vi "Helper - Overlay waypoints.vi"(11 "Refnum in":T1) -> (3 "Refnum out":T1)   [LabVIEW 2011]
uses:
  <vilib>/vision/Image Controls.llb/IMAQ Image.ctl
  2 Globals/2 Global.vi
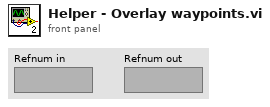
[diagram p1: front panel]
types:
  T1 = typedef "IMAQ Image.ctl" = refnum<image>
  T2 = typedef "ocuWaypoints.ctl" = cluster{"Waypoints Array":T3[], "Current Waypoint":dbl}
  T3 = typedef "ocuWaypoint.ctl" = cluster{"Point Type":T4, "Dist/Time":dbl, "UTM Location":T5}
  T4 = typedef "waypointTypes.ctl" = u16
  T5 = typedef "UTM Location.ctl" = cluster{"UTM Zone":dbl, "Hemisphere":enum16{"North", "South"}, "East":dbl, "North":dbl}
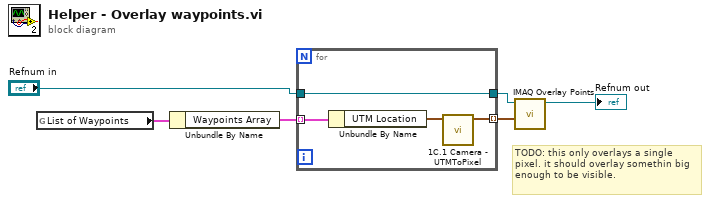
[diagram p0: block diagram]
diagram:
  # "TODO: this only overlays a single pixel. it should overlay somethin big enough to be visible."
  n1 = global read "2 Global.vi" "List of Waypoints"() -> (w2:T2)
  n2 = Unbundle By Name(w2) -> ("Waypoints Array"=w1:T3[])
  n3 = for {
    tunnel: [w7] -> w3 mode=indexing
    tunnel: "Refnum in" -> [w10]
    tunnel: [w10] -> w4
    tunnel: w1 -> [w9] mode=indexing
    n4 = Unbundle By Name(w9) -> ("UTM Location"=w8:T5)
    n5 = call "1C.1 Camera - UTMToPixel.vi"("Robot UTM Location in"=w8) -> ("output cluster"=w7:cluster{"X":i32, "Y":i32})  [unwired: 10 in]
  }
  n6 = call "IMAQ Overlay Points"("Array of Points"=w3, "Image"=w4) -> ("Image Out"=→"Refnum out":T1)  [unwired: 8 in, 1 out]
